vi "zmq_proxy.vi"(4 "error in":errorcluster, 5 "capture":refnum<class "zmq_socket.lvclass">, 6 "backend":refnum<class "zmq_socket.lvclass">, 7 "frontend":refnum<class "zmq_socket.lvclass">) -> (0 "error out":errorcluster)   [LabVIEW 2019, in "zeromq.lvlib" / "zmq_socket.lvclass"]
doc: "Starts a proxy server between the frontend and backend, with all messages passed to the capture socket, if specified. This can be used to implement a number of paradigms, such as the \"shared queue\", \"forwarder\" and \"streamer\" patterns.\n\nNote that this VI will not return until the host context is destroyed.\n\nDetailed API documentation: http://api.zeromq.org/3-2:zmq-proxy"
uses:
  zmq_socket.lvclass
  zmq_socket.lvclass/zmq_socket.ctl
  <vilib>/Utility/error.llb/Error Cluster From Error Code.vi
  zeromq.lvlib
panel:
  # "ØMQ"
  # "labview"
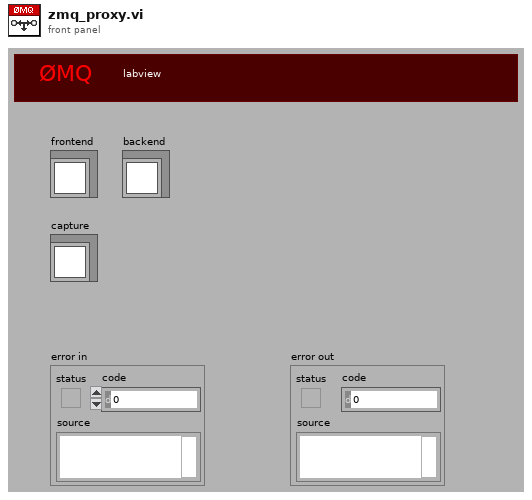
[diagram p1: front panel]
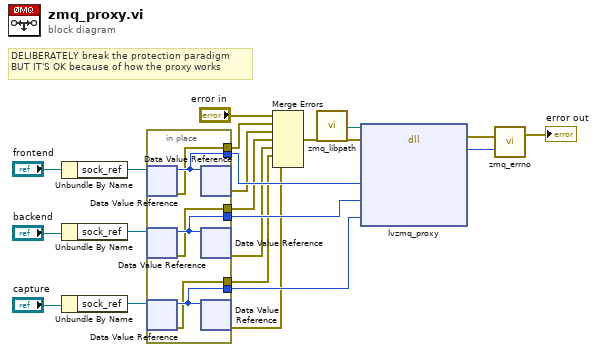
[diagram p0: block diagram]
diagram:
  # "DELIBERATELY break the protection paradigm\nBUT IT'S OK because of how the proxy works"
  n1 = Unbundle By Name("frontend") -> ("sock_ref"=w20:refnum<data-value>)
  n2 = Unbundle By Name("backend") -> ("sock_ref"=w16:refnum<data-value>)
  n3 = Unbundle By Name("capture") -> ("sock_ref"=w17:refnum<data-value>)
  n4 = in-place {
    in-place-border: [w27] -> w14
    in-place-border: [w26] -> w13
    in-place-border: [w25] -> w12
    in-place-border: [w24] -> w7
    in-place-border: [w23] -> w5
    in-place-border: [w22] -> w3
    n5 = in-place-dvr #1(w20) -> (w27:u64, w24:errorcluster)
    n6 = in-place-dvr #2(w16) -> (w26:u64, w23:errorcluster)
    n7 = in-place-dvr #3(w17) -> (w25:u64, w22:errorcluster)
    n8 = in-place-dvr #1(w27) -> (w6:errorcluster)  [unwired: 1 out]
    n9 = in-place-dvr #2(w26) -> (w4:errorcluster)  [unwired: 1 out]
    n10 = in-place-dvr #3(w25) -> (w2:errorcluster)  [unwired: 1 out]
  }
  n11 = Merge Errors("error in", w7, w6, w5, w4, w3, w2) -> (w1:errorcluster)
  n12 = call "zmq_libpath.vi"() -> ("path"=w10:path)
  n13 = dll-call lib="?" fn="lvzmq_proxy" ("zmq_labview.dll:lvzmq_socket")(path in=w10, error in=w1, "front"=w14, "back"=w13, "capture"=w12) -> (error out=w11:errorcluster, "return type"=w9:i32)  [unwired: 6 in, 1 out]
  n14 = call "zmq_errno.vi"("retval"=w9, "error in"=w11) -> ("error out"=→"error out":errorcluster)  [unwired: 1 out]
